vi "Performance Test.vi"() -> ()   [LabVIEW 2021]
uses:
  ChannelCommon/typedef/Benchmark Stats.ctl
  CIFChannels/Typedef/Direction.ctl
  ChannelCommon/typedef/FIFO Config.ctl
  CIF_NIChn_FIFO_DAQ.lvclass
  D:/dev/Packages/Channel_Manager/src/CIFChannels/CIFChannels.lvclass
  <vilib>/Platform/TimedLoop/XDataNode/timing_clust.ctl
  <vilib>/Platform/TimedLoop/XDataNode/nitl_modes.ctl
  <vilib>/Platform/TimedLoop/XDataNode/wakeup.ctl
  ChannelCommon/typedef/TimeStamps.ctl
  ChannelCommon/typedef/Datatype Waveform.ctl
  CIFChannels/CIFChannels.lvclass/CIFChannels.ctl
  <vilib>/CIF Foundation/CIF Utilities/Statistics/I64/Stats_I64_CIF_U.lvclass/Stats_I64_CIF_U.ctl
  <vilib>/CIF Foundation/CIF Utilities/DataTypes/Flatten U64.vi
  <vilib>/CIF Foundation/CIF Utilities/Statistics/I64/Get Stats.vi
  <vilib>/Platform/TimedLoop/XDataNode/XDataNode.xnode
  <vilib>/Platform/TimedLoop/XDataNode/XDNodeRunTimeDep.lvlib
  CIFChannels/CIFChannels.lvclass
  ChannelCommon/ChannelCommon.lvlib
panel:
  out "timed out? 2":bool
  out "Channel R/W (us) 2":T1
  out "Flatten (us) 2":T1
  out "Flatten (us) TO":T1
  out "Channel R/W (us) TO":T1
  out "Flatten (us)":T1
  out "Channel R/W (us)":T1
  out "avg TO":dbl
  out "max TO":dbl
  out "timed out? 3":bool
  out "timed out?":bool
  out "avg channel":dbl
  out "max channel":dbl
  out "pass":bool
  out "error out":errorcluster
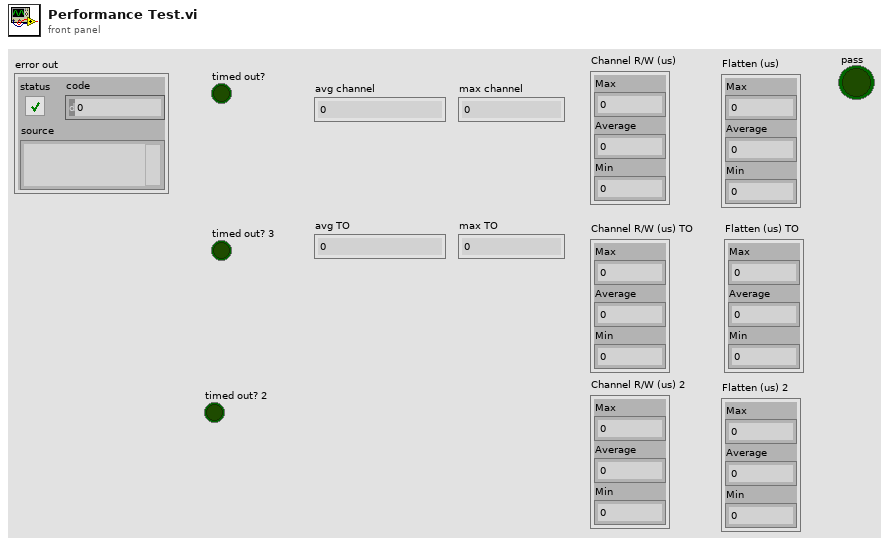
[diagram p1: front panel]
types:
  T1 = typedef "ChannelCommon.lvlib/Benchmark Stats.ctl" = cluster{"Max":i64, "Average":dbl, "Min":i64}
  T2 = typedef "ChannelCommon.lvlib/FIFO Config.ctl" = cluster{"Max Bytes/Msg":u64, "Max Msg/FIFO":u64, "Flags":u64}
  T3 = typedef "CIFChannels.lvclass/Direction.ctl" = enum16{"Publisher", "Subscriber"}
  T4 = typedef "ChannelCommon.lvlib/Datatype Waveform.ctl" = cluster{"measurement":dbl[], "dT":dbl, "Timestamp":i64, "Read Lock":bool}
  T5 = typedef "ChannelCommon.lvlib/TimeStamps.ctl" = cluster{"ClockID":u8, "T0":i64, "T_Out":i64}
  T6 = typedef "XDNodeRunTimeDep.lvlib/timing_clust.ctl" = cluster{"Expected End [f-1]":u64, "Actual End [f-1]":u64, "Finished Late? [f-1]":bool, "Expected End [i-1]":u64, "Actual End [i-1]":u64, "Finished Late? [i-1]":bool, "Expected Start [i]":u64, "Actual Start [i]":u64, "Expected Start [f]":u64, "Actual Start [f]":u64, "Source Name":string, "Structure Name":string, "Period":i64, "Deadline":i64, "Offset":i64, "Start":i64, "Priority":i32, "Timeout":i32, "Mode":T7, "Wakeup Reason":T8, "Error":errorcluster, "Source Type":string, "Secondary Source Type":string, "Global End Time":u64, "Global Start Time":u64, "Frame Duration":u64, "Iteration Duration":u64, "Assigned CPU":i32, "I/O Scan Engine Mode":u32}
  T7 = typedef "XDNodeRunTimeDep.lvlib/nitl_modes.ctl" = enum32{"No Change", "Process missed periods, maintain original phase", "Discard missed periods, maintain original phase", "Process missed periods, ignore original phase", "Discard missed periods, ignore original phase"}
  T8 = typedef "XDNodeRunTimeDep.lvlib/wakeup.ctl" = enum32{"Normal", "Aborted", "Asynchronous wakeup", "Timing source error", "Timed loop error", "Timeout"}
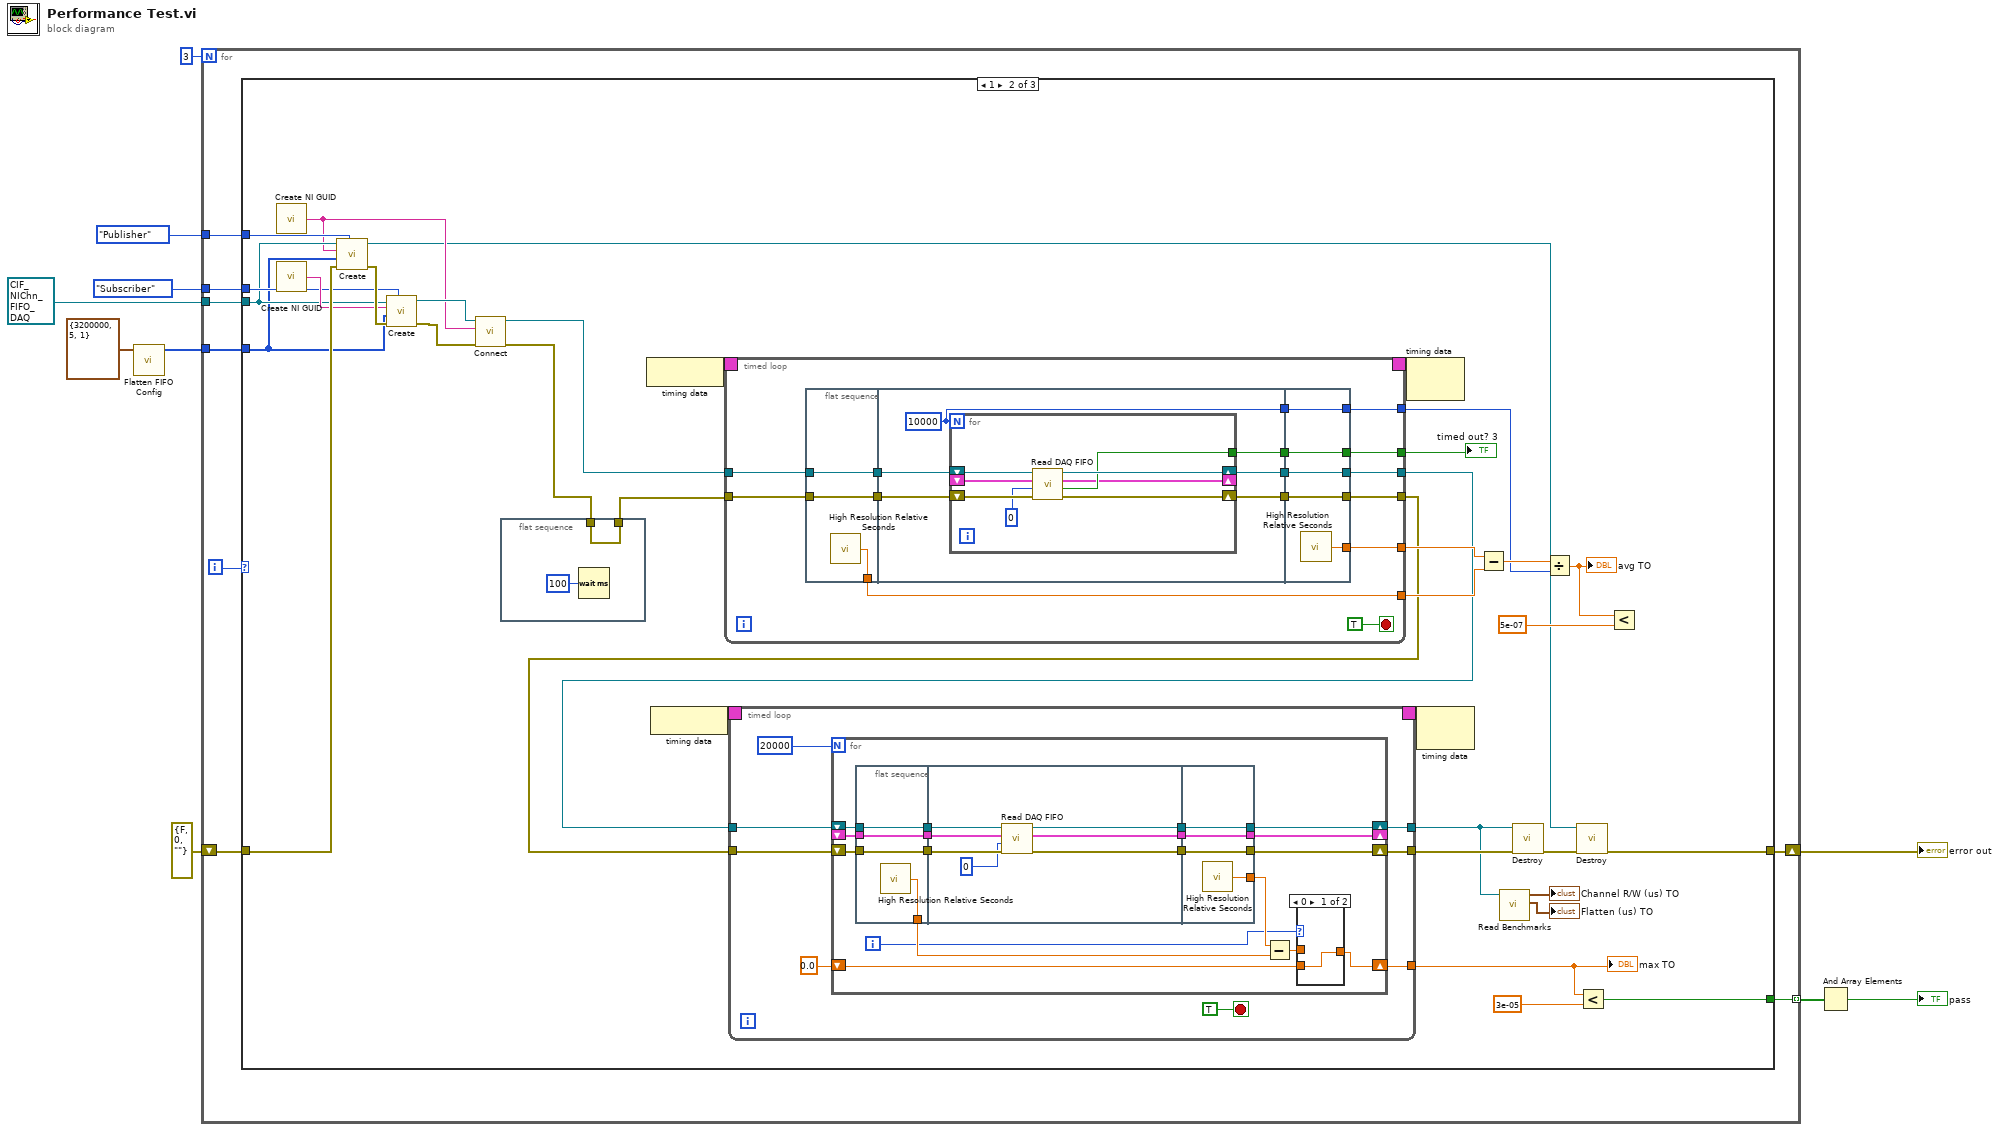
[diagram p0: block diagram]
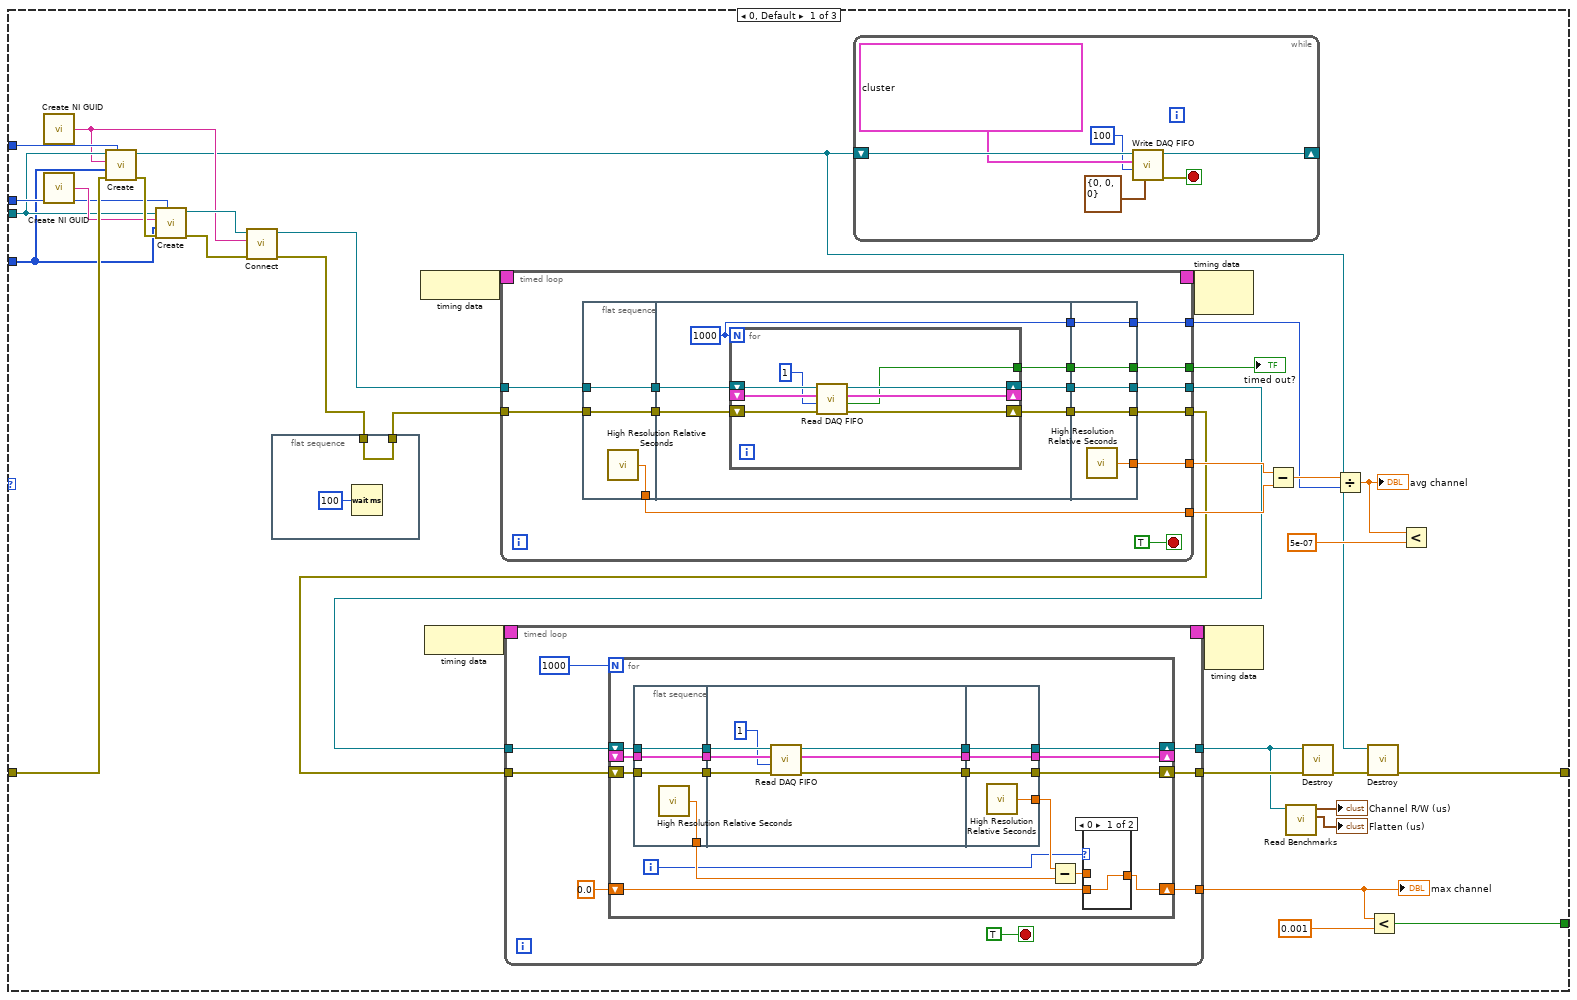
[diagram p2: hidden frame]
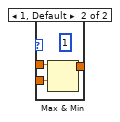
[diagram p3: hidden frame]
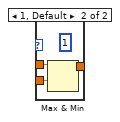
[diagram p4: hidden frame]
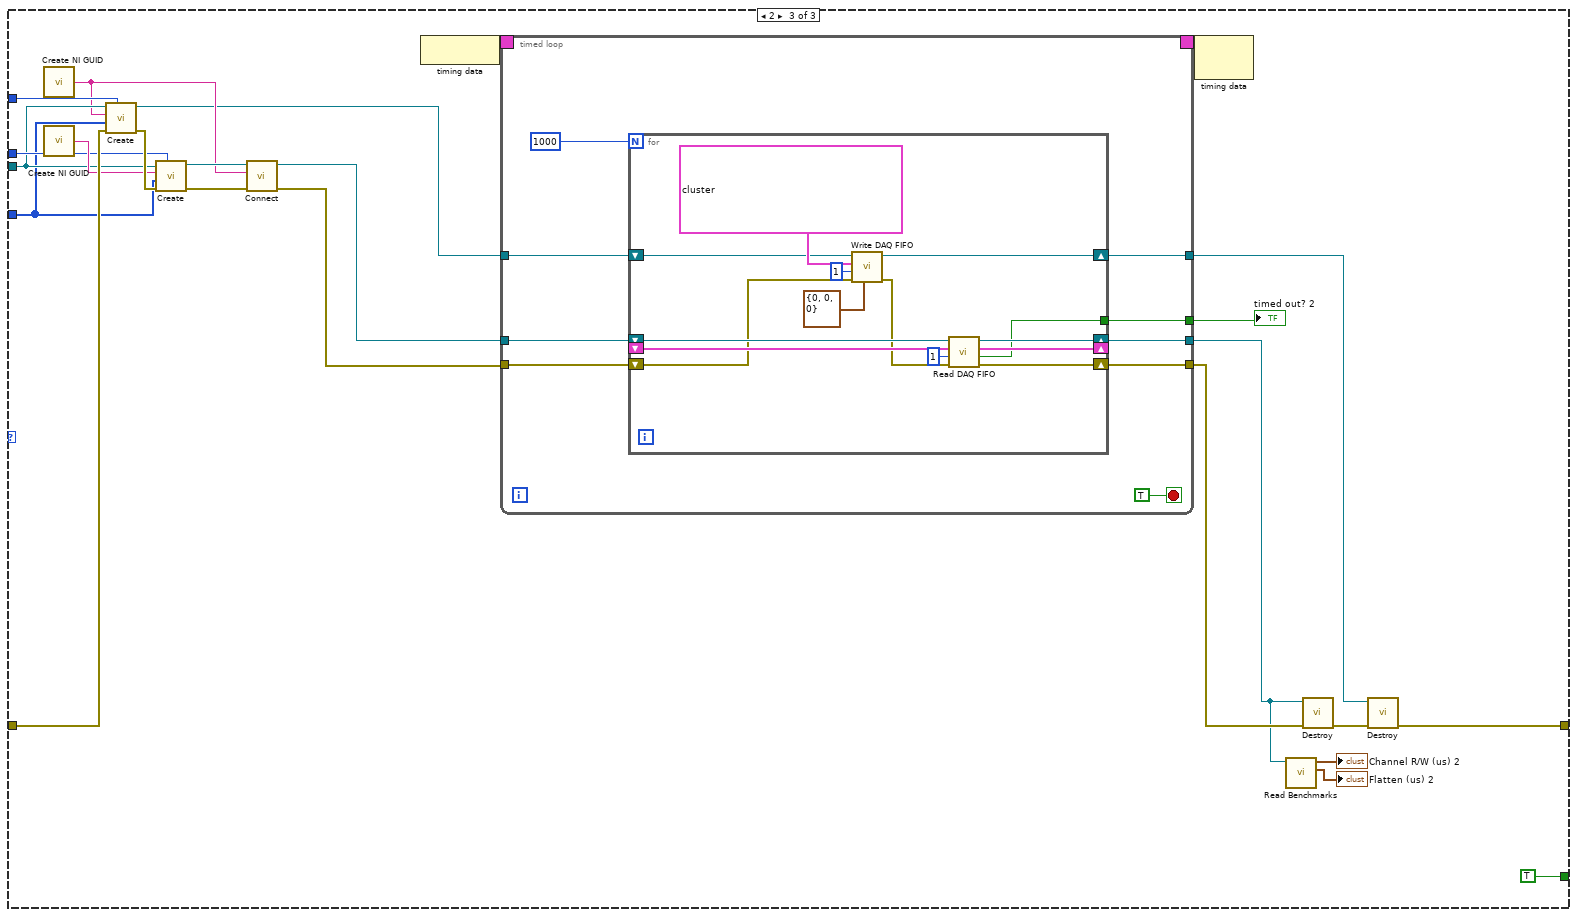
[diagram p5: hidden frame]
diagram:
  n1 = call "Flatten FIFO Config.vi"("FIFO Config in"=T2 {"Max Bytes/Msg"=3200000, "Max Msg/FIFO"=5, "Flags"=1}) -> ("Flattened FIFO Config"=w2:u8[])  [unwired: 10 in]
  n2 = for {
    N: 3 -> [_]
    tunnel: [w18] -> w8 mode=indexing
    shift-right: [w17] -> w10
    shift-left: errorcluster {"status"=FALSE, "code"=0, "source"=""} ("error out") -> [w15]
    tunnel: Direction."Publisher" ("Direction") -> [w14]
    tunnel: Direction."Subscriber" ("Direction") -> [w13]
    tunnel: refnum<class "CIF_NIChn_FIFO_DAQ.lvclass"> refnum ("CIF_NIChn_FIFO_DAQ.lvclass") -> [w12]
    tunnel: w2 -> [w11]
    i -> [w16]
    n3 = case shown="1" w16 {
      tunnel: [w40 w174 TRUE] -> w18
      tunnel: [w25 w159 w290] -> w17
      tunnel: w15 -> [w38 w172 w301]
      tunnel: w14 -> [w36 w170 w299]
      tunnel: w13 -> [w35 w169 w298]
      tunnel: w12 -> [w34 w168 w297]
      tunnel: w11 -> [w30 w164 w293]
      frame 0, Default {
        n4 = call <vilib>:"Create NI GUID.vi"() -> ("NI GUID"=w32:string)
        n5 = call <vilib>:"Create NI GUID.vi"() -> ("NI GUID"=w37:string)
        n6 = call-dynamic "Create.vi"("Direction"=w36, "error in (no error)"=w38, "Custom Config Data"=w30, "Name"=w32, "CIFFIFO in"=w34) -> ("error out"=w39:errorcluster, "CIFFIFO out"=w26:refnum<class "CIF_NIChn_FIFO_DAQ.lvclass">)  [unwired: 5 in]
        n7 = call-dynamic "Create.vi"("Direction"=w35, "error in (no error)"=w39, "Custom Config Data"=w30, "Name"=w37, "CIFFIFO in"=w34) -> ("error out"=w31:errorcluster, "CIFFIFO out"=w33:refnum<class "CIF_NIChn_FIFO_DAQ.lvclass">)  [unwired: 5 in]
        n8 = call-dynamic "Connect.vi"("error in (no error)"=w31, "Connection Name"=w32, "CIFTag in"=w33) -> ("error out"=w24:errorcluster, "CIFTag out"=w29:refnum<class "CIF_NIChn_FIFO_DAQ.lvclass">)  [unwired: 7 in]
        n9 = flat-sequence {
          tunnel: w24 -> [w56]
          tunnel: [w56] -> w23
          frame #0 {
            n10 = Wait (ms)(milliseconds to wait=u32 100) -> ()  [unwired: 1 out]
          }
        }
        n11 = node-c288() -> (w54:T6)
        n12 = node-c288() -> (w52:T6)
        n13 = timed-loop {
          timing: w54 -> [_]
          timing-out: [_] -> w53
          tunnel: w29 -> [w126]
          tunnel: w23 -> [w125]
          tunnel: [w121] -> w46
          tunnel: [w119] -> w45
          tunnel: [w117] -> w50
          tunnel: [w116] -> w49
          tunnel: [w115] -> w47
          tunnel: [w113] -> w22
          stop <- TRUE stop-if-true
          n14 = flat-sequence {
            tunnel: w125 -> [w128]
            tunnel: w126 -> [w129]
            tunnel: [w129] -> w123
            tunnel: [w128] -> w122
            tunnel: [w127] -> w116
            tunnel: w123 -> [w135]
            tunnel: w122 -> [w134]
            tunnel: [w133] -> w120
            tunnel: [w132] -> w118
            tunnel: [w131] -> w114
            tunnel: [w130] -> w112
            tunnel: [w148] -> w121
            tunnel: w120 -> [w148]
            tunnel: [w147] -> w119
            tunnel: w118 -> [w147]
            tunnel: [w146] -> w117
            tunnel: [w145] -> w115
            tunnel: w114 -> [w145]
            tunnel: [w144] -> w113
            tunnel: w112 -> [w144]
            frame #0 {
              n15 = call <vilib>:"High Resolution Relative Seconds.vi"() -> ("relative seconds"=w127:dbl)
            }
            frame #1 {
              w131 = 1000
              n16 = for {
                N: w131 -> [_]
                shift-right: [w138] -> w133
                shift-left: w135 -> [w143]
                shift-right: [w141] -> w132
                shift-left: w134 -> [w142]
                shift-right: [w140] -> _
                shift-left: _ -> [w139]
                tunnel: [w137] -> w130
                n17 = call-dynamic "Read DAQ FIFO.vi"("error in (no error)"=w142, "Timeout (ms)"=1, "Data In"=w139, "CIF_NIChn_FIFO_DAQ in"=w143) -> ("error out"=w141:errorcluster, "timed out?"=w137:bool, "Data Out"=w140:T4[], "CIF_NIChn_FIFO_DAQ out"=w138:refnum<class "CIF_NIChn_FIFO_DAQ.lvclass">)  [unwired: 3 in, 1 out]
              }
            }
            frame #2 {
              n18 = call <vilib>:"High Resolution Relative Seconds.vi"() -> ("relative seconds"=w146:dbl)
            }
          }
        }
        "timed out?" <- w22
        n19 = timed-loop {
          timing: w52 -> [_]
          timing-out: [_] -> w51
          tunnel: w46 -> [w70]
          tunnel: w45 -> [w69]
          tunnel: [w67] -> w21
          tunnel: [w66] -> w28
          tunnel: [w63] -> w42
          stop <- TRUE stop-if-true
          n20 = for {
            N: 1000 -> [_]
            shift-right: [w82] -> w67
            shift-left: w70 -> [w84]
            shift-right: [w81] -> w66
            shift-left: w69 -> [w83]
            shift-right: [w75] -> w63
            shift-left: 0.0 -> [w76]
            shift-right: [w74] -> _
            shift-left: _ -> [w80]
            i -> [w72]
            n21 = flat-sequence {
              tunnel: w83 -> [w95]
              tunnel: w84 -> [w96]
              tunnel: [w96] -> w88
              tunnel: [w95] -> w87
              tunnel: [w94] -> w78
              tunnel: w80 -> [w93]
              tunnel: [w93] -> w86
              tunnel: w88 -> [w103]
              tunnel: w87 -> [w102]
              tunnel: [w99] -> w85
              tunnel: w86 -> [w98]
              tunnel: [w100] -> w73
              tunnel: [w101] -> w71
              tunnel: [w107] -> w82
              tunnel: w85 -> [w107]
              tunnel: [w106] -> w81
              tunnel: [w105] -> w79
              tunnel: [w104] -> w74
              tunnel: w73 -> [w104]
              tunnel: w71 -> [w106]
              frame #0 {
                n22 = call <vilib>:"High Resolution Relative Seconds.vi"() -> ("relative seconds"=w94:dbl)
              }
              frame #1 {
                n23 = call-dynamic "Read DAQ FIFO.vi"("error in (no error)"=w102, "Timeout (ms)"=1, "Data In"=w98, "CIF_NIChn_FIFO_DAQ in"=w103) -> ("error out"=w101:errorcluster, "Data Out"=w100:T4[], "CIF_NIChn_FIFO_DAQ out"=w99:refnum<class "CIF_NIChn_FIFO_DAQ.lvclass">)  [unwired: 3 in, 2 out]
              }
              frame #2 {
                n24 = call <vilib>:"High Resolution Relative Seconds.vi"() -> ("relative seconds"=w105:dbl)
              }
            }
            n25 = Subtract(x=w79, y=w78) -> (x-y=w77:dbl)
            n26 = case shown="0" w72 {
              tunnel: w77 -> [_ w92]
              tunnel: w76 -> [w89 w91]
              tunnel: [w89 w90] -> w75
              frame 0 {
              }
              frame 1, Default {
                (unwired) u32 1 ("milliseconds to wait")
                n27 = Max & Min(x=w92, y=w91) -> (max(x,y)=w90:dbl)  [unwired: 1 out]
              }
            }
          }
        }
        "max channel" <- w42
        n28 = while {
          shift-right: [w59] -> _
          shift-left: w26 -> [w62]
          stop <- w60 stop-if-true
          n29 = call-dynamic "Write DAQ FIFO.vi"("FIFO Timestamps"=T5 {"ClockID"=0, "T0"=0, "T_Out"=0}, "Timeout (ms)"=100, "Data In"=T4[] [{"measurement"=array[200001 elements], "dT"=43.0, "Timestamp"=2, "Read Lock"=FALSE}, {"measurement"=array[200001 elements], "dT"=34.0, "Timestamp"=1, "Read Lock"=FALSE}] ("DAQ In"), "CIF_NIChn_FIFO_DAQ in"=w62) -> ("error out"=w60:errorcluster, "CIF_NIChn_FIFO_DAQ out"=w59:refnum<class "CIF_NIChn_FIFO_DAQ.lvclass">)  [unwired: 4 in, 2 out]
        }
        n30 = node-c288(w53) -> ()  [unwired: 1 out]
        n31 = node-c288(w51) -> ()  [unwired: 1 out]
        n32 = Subtract(x=w50, y=w49) -> (x-y=w48:dbl)
        n33 = call "Read Benchmarks.vi"("CIFChannels in"=w21) -> ("Flatten (us)"=→"Flatten (us)":T1, "Channel R/W (us)"=→"Channel R/W (us)":T1)  [unwired: 9 in]
        n34 = call-dynamic "Destroy.vi"("error in (no error)"=w28, "CIFFIFO in"=w21) -> ("error out"=w27:errorcluster)  [unwired: 8 in, 1 out]
        n35 = Divide(x=w48, y=w47) -> (x/y=w44:dbl)
        "avg channel" <- w44
        n36 = call-dynamic "Destroy.vi"("error in (no error)"=w27, "CIFFIFO in"=w26) -> ("error out"=w25:errorcluster)  [unwired: 8 in, 1 out]
        n37 = Less?(x=w42, y=0.001) -> (x < y?=w40:bool)
        n38 = Less?(x=w44, y=5e-07) -> ()  [unwired: 1 out]
      }
      frame 1 {
        n39 = call <vilib>:"Create NI GUID.vi"() -> ("NI GUID"=w166:string)
        n40 = call <vilib>:"Create NI GUID.vi"() -> ("NI GUID"=w171:string)
        n41 = call-dynamic "Create.vi"("Direction"=w170, "error in (no error)"=w172, "Custom Config Data"=w164, "Name"=w166, "CIFFIFO in"=w168) -> ("error out"=w173:errorcluster, "CIFFIFO out"=w160:refnum<class "CIF_NIChn_FIFO_DAQ.lvclass">)  [unwired: 5 in]
        n42 = call-dynamic "Create.vi"("Direction"=w169, "error in (no error)"=w173, "Custom Config Data"=w164, "Name"=w171, "CIFFIFO in"=w168) -> ("error out"=w165:errorcluster, "CIFFIFO out"=w167:refnum<class "CIF_NIChn_FIFO_DAQ.lvclass">)  [unwired: 5 in]
        n43 = call-dynamic "Connect.vi"("error in (no error)"=w165, "Connection Name"=w166, "CIFTag in"=w167) -> ("error out"=w158:errorcluster, "CIFTag out"=w163:refnum<class "CIF_NIChn_FIFO_DAQ.lvclass">)  [unwired: 7 in]
        n44 = flat-sequence {
          tunnel: w158 -> [w190]
          tunnel: [w190] -> w157
          frame #0 {
            n45 = Wait (ms)(milliseconds to wait=u32 100) -> ()  [unwired: 1 out]
          }
        }
        n46 = node-c288() -> (w188:T6)
        n47 = node-c288() -> (w186:T6)
        n48 = timed-loop {
          timing: w188 -> [_]
          timing-out: [_] -> w187
          tunnel: w163 -> [w254]
          tunnel: w157 -> [w253]
          tunnel: [w249] -> w180
          tunnel: [w247] -> w179
          tunnel: [w245] -> w184
          tunnel: [w244] -> w183
          tunnel: [w243] -> w181
          tunnel: [w241] -> w156
          stop <- TRUE stop-if-true
          n49 = flat-sequence {
            tunnel: w253 -> [w256]
            tunnel: w254 -> [w257]
            tunnel: [w257] -> w251
            tunnel: [w256] -> w250
            tunnel: [w255] -> w244
            tunnel: w251 -> [w263]
            tunnel: w250 -> [w262]
            tunnel: [w261] -> w248
            tunnel: [w260] -> w246
            tunnel: [w259] -> w242
            tunnel: [w258] -> w240
            tunnel: [w276] -> w249
            tunnel: w248 -> [w276]
            tunnel: [w275] -> w247
            tunnel: w246 -> [w275]
            tunnel: [w274] -> w245
            tunnel: [w273] -> w243
            tunnel: w242 -> [w273]
            tunnel: [w272] -> w241
            tunnel: w240 -> [w272]
            frame #0 {
              n50 = call <vilib>:"High Resolution Relative Seconds.vi"() -> ("relative seconds"=w255:dbl)
            }
            frame #1 {
              w259 = 10000
              n51 = for {
                N: w259 -> [_]
                shift-right: [w268] -> w261
                shift-left: w263 -> [w271]
                shift-right: [w269] -> w260
                shift-left: w262 -> [w270]
                shift-right: [w266] -> _
                shift-left: _ -> [w265]
                tunnel: [w267] -> w258
                n52 = call-dynamic "Read DAQ FIFO.vi"("error in (no error)"=w270, "Timeout (ms)"=0, "Data In"=w265, "CIF_NIChn_FIFO_DAQ in"=w271) -> ("error out"=w269:errorcluster, "timed out?"=w267:bool, "Data Out"=w266:T4[], "CIF_NIChn_FIFO_DAQ out"=w268:refnum<class "CIF_NIChn_FIFO_DAQ.lvclass">)  [unwired: 3 in, 1 out]
              }
            }
            frame #2 {
              n53 = call <vilib>:"High Resolution Relative Seconds.vi"() -> ("relative seconds"=w274:dbl)
            }
          }
        }
        "timed out? 3" <- w156
        n54 = timed-loop {
          timing: w186 -> [_]
          timing-out: [_] -> w185
          tunnel: w180 -> [w198]
          tunnel: w179 -> [w197]
          tunnel: [w195] -> w153
          tunnel: [w194] -> w162
          tunnel: [w191] -> w176
          stop <- TRUE stop-if-true
          n55 = for {
            N: 20000 -> [_]
            shift-right: [w210] -> w195
            shift-left: w198 -> [w212]
            shift-right: [w209] -> w194
            shift-left: w197 -> [w211]
            shift-right: [w203] -> w191
            shift-left: 0.0 -> [w204]
            shift-right: [w202] -> _
            shift-left: _ -> [w208]
            i -> [w200]
            n56 = flat-sequence {
              tunnel: w211 -> [w223]
              tunnel: w212 -> [w224]
              tunnel: [w224] -> w216
              tunnel: [w223] -> w215
              tunnel: [w222] -> w206
              tunnel: w208 -> [w221]
              tunnel: [w221] -> w214
              tunnel: w216 -> [w231]
              tunnel: w215 -> [w227]
              tunnel: [w230] -> w213
              tunnel: w214 -> [w228]
              tunnel: [w229] -> w201
              tunnel: [w226] -> w199
              tunnel: [w235] -> w210
              tunnel: w213 -> [w235]
              tunnel: [w234] -> w209
              tunnel: [w233] -> w207
              tunnel: [w232] -> w202
              tunnel: w201 -> [w232]
              tunnel: w199 -> [w234]
              frame #0 {
                n57 = call <vilib>:"High Resolution Relative Seconds.vi"() -> ("relative seconds"=w222:dbl)
              }
              frame #1 {
                n58 = call-dynamic "Read DAQ FIFO.vi"("error in (no error)"=w227, "Timeout (ms)"=0, "Data In"=w228, "CIF_NIChn_FIFO_DAQ in"=w231) -> ("error out"=w226:errorcluster, "Data Out"=w229:T4[], "CIF_NIChn_FIFO_DAQ out"=w230:refnum<class "CIF_NIChn_FIFO_DAQ.lvclass">)  [unwired: 3 in, 2 out]
              }
              frame #2 {
                n59 = call <vilib>:"High Resolution Relative Seconds.vi"() -> ("relative seconds"=w233:dbl)
              }
            }
            n60 = Subtract(x=w207, y=w206) -> (x-y=w205:dbl)
            n61 = case shown="0" w200 {
              tunnel: w205 -> [_ w220]
              tunnel: w204 -> [w217 w219]
              tunnel: [w217 w218] -> w203
              frame 0 {
              }
              frame 1, Default {
                (unwired) u32 1 ("milliseconds to wait")
                n62 = Max & Min(x=w220, y=w219) -> (max(x,y)=w218:dbl)  [unwired: 1 out]
              }
            }
          }
        }
        "max TO" <- w176
        n63 = node-c288(w187) -> ()  [unwired: 1 out]
        n64 = node-c288(w185) -> ()  [unwired: 1 out]
        n65 = Subtract(x=w184, y=w183) -> (x-y=w182:dbl)
        n66 = call "Read Benchmarks.vi"("CIFChannels in"=w153) -> ("Flatten (us)"=→"Flatten (us) TO":T1, "Channel R/W (us)"=→"Channel R/W (us) TO":T1)  [unwired: 9 in]
        n67 = call-dynamic "Destroy.vi"("error in (no error)"=w162, "CIFFIFO in"=w153) -> ("error out"=w161:errorcluster)  [unwired: 8 in, 1 out]
        n68 = Divide(x=w182, y=w181) -> (x/y=w178:dbl)
        "avg TO" <- w178
        n69 = call-dynamic "Destroy.vi"("error in (no error)"=w161, "CIFFIFO in"=w160) -> ("error out"=w159:errorcluster)  [unwired: 8 in, 1 out]
        n70 = Less?(x=w176, y=3e-05) -> (x < y?=w174:bool)
        n71 = Less?(x=w178, y=5e-07) -> ()  [unwired: 1 out]
      }
      frame 2 {
        n72 = call <vilib>:"Create NI GUID.vi"() -> ("NI GUID"=w295:string)
        n73 = call <vilib>:"Create NI GUID.vi"() -> ("NI GUID"=w300:string)
        n74 = call-dynamic "Create.vi"("Direction"=w299, "error in (no error)"=w301, "Custom Config Data"=w293, "Name"=w295, "CIFFIFO in"=w297) -> ("error out"=w302:errorcluster, "CIFFIFO out"=w286:refnum<class "CIF_NIChn_FIFO_DAQ.lvclass">)  [unwired: 5 in]
        n75 = call-dynamic "Create.vi"("Direction"=w298, "error in (no error)"=w302, "Custom Config Data"=w293, "Name"=w300, "CIFFIFO in"=w297) -> ("error out"=w294:errorcluster, "CIFFIFO out"=w296:refnum<class "CIF_NIChn_FIFO_DAQ.lvclass">)  [unwired: 5 in]
        n76 = call-dynamic "Connect.vi"("error in (no error)"=w294, "Connection Name"=w295, "CIFTag in"=w296) -> ("error out"=w282:errorcluster, "CIFTag out"=w292:refnum<class "CIF_NIChn_FIFO_DAQ.lvclass">)  [unwired: 7 in]
        n77 = node-c288() -> (w304:T6)
        n78 = timed-loop {
          timing: w304 -> [_]
          timing-out: [_] -> w303
          tunnel: w292 -> [w313]
          tunnel: w282 -> [w312]
          tunnel: [w310] -> w283
          tunnel: [w309] -> w284
          tunnel: [w307] -> w289
          tunnel: w286 -> [w306]
          tunnel: [w305] -> w285
          stop <- TRUE stop-if-true
          n79 = for {
            N: 1000 -> [_]
            shift-right: [w323] -> w310
            shift-left: w313 -> [w327]
            shift-right: [w326] -> w309
            shift-left: w312 -> [w319]
            shift-right: [w325] -> _
            shift-left: _ -> [w324]
            tunnel: [w322] -> w307
            shift-right: [w316] -> w305
            shift-left: w306 -> [w317]
            n80 = call-dynamic "Write DAQ FIFO.vi"("FIFO Timestamps"=T5 {"ClockID"=0, "T0"=0, "T_Out"=0}, "error in (no error)"=w319, "Timeout (ms)"=1, "Data In"=T4[] [{"measurement"=array[200001 elements], "dT"=43.0, "Timestamp"=2, "Read Lock"=FALSE}, {"measurement"=array[200001 elements], "dT"=34.0, "Timestamp"=1, "Read Lock"=FALSE}] ("DAQ In"), "CIF_NIChn_FIFO_DAQ in"=w317) -> ("error out"=w318:errorcluster, "CIF_NIChn_FIFO_DAQ out"=w316:refnum<class "CIF_NIChn_FIFO_DAQ.lvclass">)  [unwired: 3 in, 2 out]
            n81 = call-dynamic "Read DAQ FIFO.vi"("error in (no error)"=w318, "Timeout (ms)"=1, "Data In"=w324, "CIF_NIChn_FIFO_DAQ in"=w327) -> ("error out"=w326:errorcluster, "timed out?"=w322:bool, "Data Out"=w325:T4[], "CIF_NIChn_FIFO_DAQ out"=w323:refnum<class "CIF_NIChn_FIFO_DAQ.lvclass">)  [unwired: 3 in, 1 out]
          }
        }
        "timed out? 2" <- w289
        n82 = node-c288(w303) -> ()  [unwired: 1 out]
        n83 = call "Read Benchmarks.vi"("CIFChannels in"=w283) -> ("Flatten (us)"=→"Flatten (us) 2":T1, "Channel R/W (us)"=→"Channel R/W (us) 2":T1)  [unwired: 9 in]
        n84 = call-dynamic "Destroy.vi"("error in (no error)"=w284, "CIFFIFO in"=w283) -> ("error out"=w291:errorcluster)  [unwired: 8 in, 1 out]
        n85 = call-dynamic "Destroy.vi"("error in (no error)"=w291, "CIFFIFO in"=w285) -> ("error out"=w290:errorcluster)  [unwired: 8 in, 1 out]
      }
    }
  }
  "error out" <- w10
  n86 = And Array Elements(Boolean array=w8) -> (logical AND=→"pass":bool)
